vi "sub_pf_motion-model.vi"(10 "u":T1, 11 "x_true":T1) -> (3 "x_true out":T1)   [LabVIEW 2019]
uses:
  <vilib>/Analysis/Matrix/Datatypes/RealMatrix.ctl
  Ctrl/cmd_common.ctl
  <vilib>/Analysis/Matrix/Numeric/Multiply/Multiply - RM,RM.vi
  <vilib>/Analysis/Matrix/Numeric/Add/Add - RM,RM.vi
  <vilib>/Analysis/Matrix/NI_Matrix.lvlib
panel:
  out "행 x_true":i32
  out "열 x_true":i32
  out "열 F":i32
  out "행 F":i32
  out "B":T1
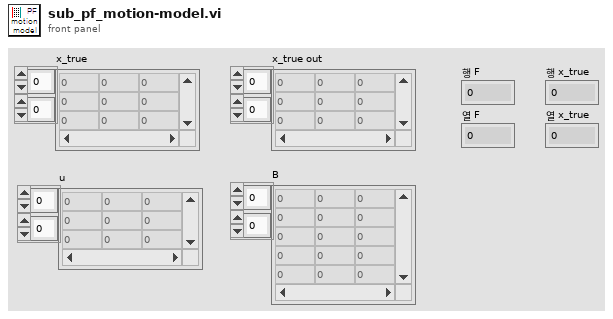
[diagram p1: front panel]
types:
  T1 = typedef "NI_Matrix.lvlib/RealMatrix.ctl" = dbl[][]
  T2 = typedef "cmd_common.ctl" = enum16{"read", "write"}
  T3 = cluster{"DT":dbl, "SIM_TIME":dbl, "MAX_RANGE":dbl, "NP":u32, "NTh":u32, "Q":T1, "R":T1, "Q_sim":T1, "R_sim":T1, "rf_id":cluster{"x":dbl, "y":dbl}[]}
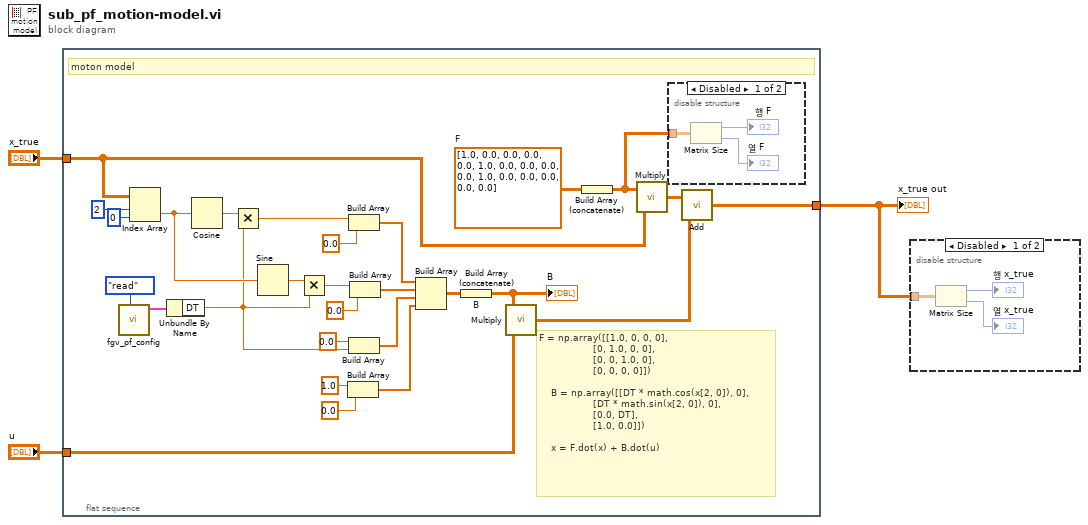
[diagram p0: block diagram]
diagram:
  n1 = flat-sequence {
    tunnel: "x_true" -> [w11]
    tunnel: "u" -> [w9]
    tunnel: [w5] -> w1
    frame #0 {
      w12 = dbl[][] [[1.0, 0.0, 0.0, 0.0], [0.0, 1.0, 0.0, 0.0], [0.0, 0.0, 1.0, 0.0], [0.0, 0.0, 0.0, 0.0]]  # F
      # "F = np.array([[1.0, 0, 0, 0],\n                  [0, 1.0, 0, 0],\n                  [0, 0, 1.0, 0],\n                  [0, 0, 0, 0]])\n\n    B = np.array([[DT * math.cos(x[2, 0]), 0],\n                  [DT * math.sin(x[2, 0]), 0],\n                  [0.0, DT],\n                  [1.0, 0.0]])\n\n    x = F.dot(x) + B.dot(u)"
      # "moton model"
      n2 = call "fgv_pf_config.vi"("cmd"=cmd_common."read") -> ("pf-val out"=w7:T3)  [unwired: 10 in]
      n3 = Index Array(array=w11, index (row)=2 ("인덱스 (행)"), index (col)=0 ("인덱스 (열)")) -> (element=w27:dbl)
      n4 = Unbundle By Name(w7) -> ("DT"=w6:dbl)
      n5 = Cosine(x=w27) -> (cos(x)=w29:dbl)
      n6 = Multiply(x=w29, y=w6) -> (x*y=w26:dbl)
      n7 = Sine(x=w27) -> (sin(x)=w28:dbl)
      n8 = Multiply(x=w28, y=w6) -> (x*y=w23:dbl)
      n9 = Build Array(1.0 ("원소"), 0.0 ("원소")) -> (w19:dbl[])
      n10 = Build Array(w26, 0.0 ("원소")) -> (w16:dbl[])
      n11 = Build Array(0.0 ("원소"), w6) -> (w18:dbl[])
      n12 = Build Array(w23, 0.0 ("원소")) -> (w17:dbl[])
      n13 = Build Array(w16, w17, w18, w19) -> (w15:dbl[][])
      n14 = Build Array (concatenate) "B"(w15) -> (w14:T1)
      "B" <- w14
      n15 = call-poly <vilib>:"Multiply.vi"("Real Matrix B"=w9, "Real Matrix A"=w14) -> ("A * B"=w13:T1)
      n16 = Build Array (concatenate)(w12) -> (w4:T1)
      n17 = call-poly <vilib>:"Multiply.vi"("Real Matrix B"=w11, "Real Matrix A"=w4) -> ("A * B"=w10:T1)
      n18 = disable-structure shown="Disabled" {
        disable-tunnel: w4 -> [w34 _]
        frame Disabled {
          n19 = Matrix Size(0:w34) -> (1:→"행 F":i32, 2:→"열 F":i32)
        }
        frame Enabled {
        }
      }
      n20 = call-poly <vilib>:"Add.vi"("Real Matrix B"=w13, "Real Matrix A"=w10) -> ("A + B"=w5:T1)
    }
  }
  n21 = disable-structure shown="Disabled" {
    disable-tunnel: w1 -> [w35 _]
    frame Disabled {
      n22 = Matrix Size(0:w35) -> (1:→"행 x_true":i32, 2:→"열 x_true":i32)
    }
    frame Enabled {
    }
  }
  "x_true out" <- w1
